vi "date convertion back to 24 hour clock.vi"(11 "DateTime as string":string) -> (2 "Time":string, 3 "Date":string)   [LabVIEW 2010]
uses:
  <vilib>/Utility/miscctls.llb/LVDateTimeRec.ctl
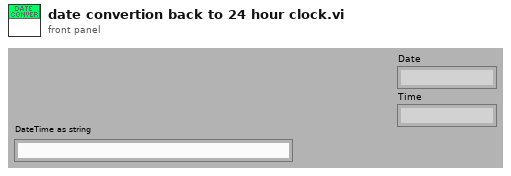
[diagram p1: front panel]
types:
  T1 = typedef "LVDateTimeRec.ctl" = cluster{"fractional second":dbl, "second":i32, "minute":i32, "hour":i32, "day of month":i32, "month":i32, "year":i32, "day of week":i32, "day of year":i32, "DST":i32}
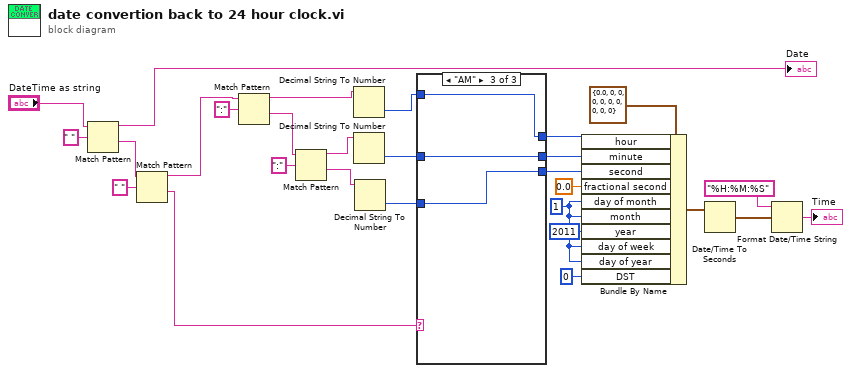
[diagram p0: block diagram]
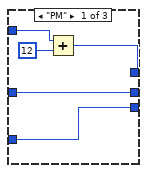
[diagram p2: hidden frame]
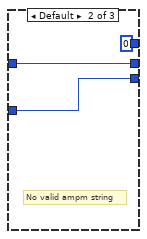
[diagram p3: hidden frame]
diagram:
  w1 = 1 ("day of month")
  n1 = Match Pattern(string="DateTime as string", regular expression=" ") -> (before substring=→"Date":string, after substring=w20:string)  [unwired: 1 in, 2 out]
  n2 = Match Pattern(string=w20, regular expression=" ") -> (before substring=w15:string, after substring=w18:string)  [unwired: 1 in, 2 out]
  n3 = Match Pattern(string=w15, regular expression=":") -> (before substring=w14:string, after substring=w13:string)  [unwired: 1 in, 2 out]
  n4 = Match Pattern(string=w13, regular expression=":") -> (before substring=w12:string, after substring=w7:string)  [unwired: 1 in, 2 out]
  n5 = Decimal String To Number(string=w14) -> (number=w10:i32)  [unwired: 2 in, 1 out]
  n6 = Decimal String To Number(string=w12) -> (number=w8:i32)  [unwired: 2 in, 1 out]
  n7 = Decimal String To Number(string=w7) -> (number=w6:i32)  [unwired: 2 in, 1 out]
  n8 = case shown="\"AM\"" w18 {
    tunnel: w10 -> [w33 _ w39]
    tunnel: [w31 0 ("offset past number") w39] -> w11
    tunnel: w8 -> [w30 w35 w38]
    tunnel: [w30 w35 w38] -> w9
    tunnel: w6 -> [w29 w34 w37]
    tunnel: [w29 w34 w37] -> w5
    frame "PM" {
      n9 = Add(x=w33, y=12) -> (x+y=w31:i32)
    }
    frame Default {
      # "No valid ampm string"
    }
    frame "AM" {
    }
  }
  n10 = Bundle By Name(cluster=T1 {"fractional second"=0.0, "second"=0, "minute"=0, "hour"=0, "day of month"=0, "month"=0, "year"=0, "day of week"=0, "day of year"=0, "DST"=0} ("date time rec"), "hour"=w11, "minute"=w9, "second"=w5, "fractional second"=0.0, "day of month"=w1, "month"=w1, "year"=2011, "day of week"=w1, "day of year"=w1, "DST"=0) -> (w27:T1)
  n11 = Date/Time To Seconds(2:w27) -> (0:w26:timestamp)  [unwired: 1 in]
  n12 = Format Date/Time String(time format string (%c)="%H:%M:%S", seconds (now)=w26) -> (date/time string=→"Time":string)  [unwired: 1 in]
